vi "Timestamp To String.vi"(5 "Formatting (auto)":string, 8 "error in (no error)":errorcluster, 10 "Time Stamp":timestamp, 11 "Registry Object":refnum<class "Carya Config.lvclass">) -> (0 "error out":errorcluster, 2 "String":string, 3 "Registry Object":refnum<class "Carya Config.lvclass">)   [LabVIEW 2013, in "Carya Config.lvclass"]
doc: "Copyright 2018, Carya Automatisering, Wiebe Walstra."
uses:
  Carya Config.lvclass
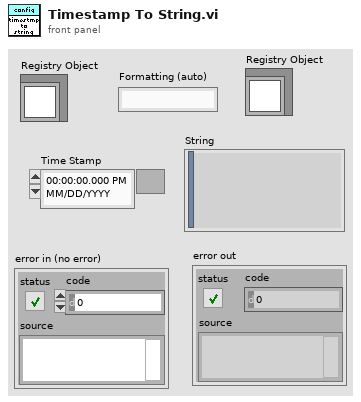
[diagram p1: front panel]
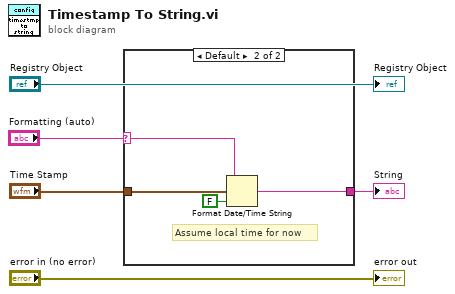
[diagram p0: block diagram]
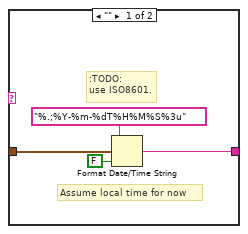
[diagram p2: hidden frame]
diagram:
  n1 = case shown="Default" "Formatting (auto)" {
    selector: "Formatting (auto)" -> [_ w10]
    tunnel: "Time Stamp" -> [w9 w13]
    tunnel: [w6 w11] -> w2
    frame "" {
      # ":TODO:\nuse ISO8601."
      # "Assume local time for now"
      n2 = Format Date/Time String(time format string (%c)="%.;%Y-%m-%dT%H%M%S%3u", seconds (now)=w9, UTC format=FALSE) -> (date/time string=w6:string)
    }
    frame Default {
      # "Assume local time for now"
      n3 = Format Date/Time String(time format string (%c)=w10, seconds (now)=w13, UTC format=FALSE) -> (date/time string=w11:string)
    }
  }
  "String" <- w2
  "Registry Object" <- "Registry Object"
  "error out" <- "error in (no error)"
